vi "Build Board Map.vi"(1 "Map":string="        ...#\n        .#..\n        #...\n        ....\n...#.......#\n........#...\n..#....#....\n..........#.\n        ...#....\n        .....#..\n        .#......\n        ......#.") -> (0 "Board Map":T1[][](array[typedef]) items=["Empty", "Portal", "Open", "Wall", ">", "<", ">-^", ">-v", "^-<", "v-<"])   [LabVIEW 2020, in "AoC 2022.lvlib"]
uses:
  AoC 2022.lvlib
  Map Tile.ctl
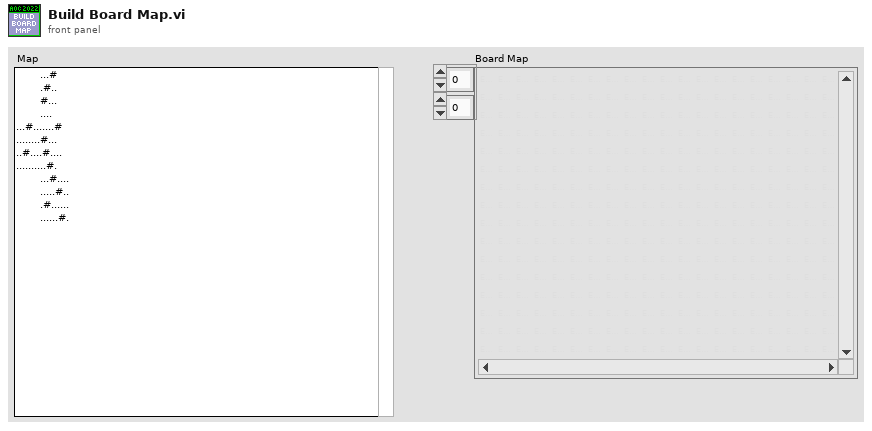
[diagram p1: front panel]
types:
  T1 = typedef "AoC 2022.lvlib/Map Tile.ctl" = u16
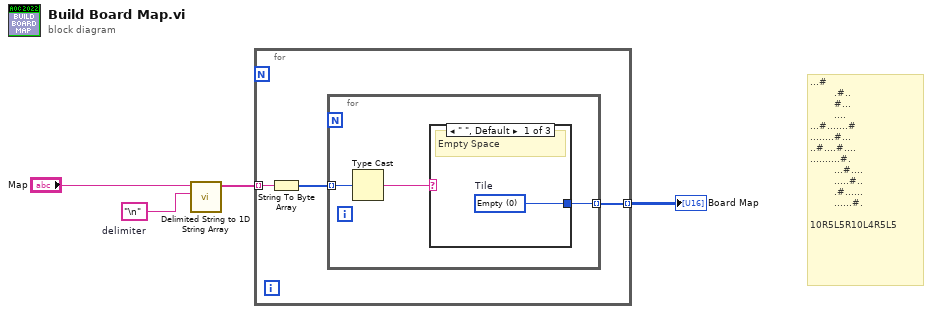
[diagram p0: block diagram]
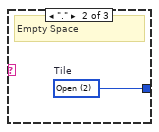
[diagram p2: hidden frame]
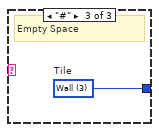
[diagram p3: hidden frame]
diagram:
  w2 = "\n"  # delimiter
  # "...#\n        .#..\n        #...\n        ....\n...#.......#\n........#...\n..#....#....\n..........#.\n        ...#....\n        .....#..\n        .#......\n        ......#.\n\n10R5L5R10L4R5L5"
  n1 = call <vilib>:"Delimited String to 1D String Array.vi"("delimiter"=w2, "delimited string"="Map") -> ("string array"=w3:string[])  [unwired: 9 in]
  n2 = for {
    tunnel: w3 -> [w7] mode=indexing
    tunnel: [w5] -> w4 mode=indexing
    n3 = String To Byte Array(string=w7) -> (unsigned byte array=w6:u8[])
    n4 = for {
      tunnel: w6 -> [w10] mode=indexing
      tunnel: [w8] -> w5 mode=indexing
      n5 = Type Cast(x=w10) -> (*(type *) &x=w9:string)  [unwired: 1 in]
      n6 = case shown="\" \", Default" w9 {
        tunnel: [w11 w12 w13] -> w8
        frame " ", Default {
          w11 = T1 0 items=["Empty", "Portal", "Open", "Wall", ">", "<", ">-^", ">-v", "^-<", "v-<"]  # Tile
          # "Empty Space"
        }
        frame "." {
          w12 = T1 2 items=["Empty", "Portal", "Open", "Wall", ">", "<", ">-^", ">-v", "^-<", "v-<"]  # Tile
          # "Empty Space"
        }
        frame "#" {
          w13 = T1 3 items=["Empty", "Portal", "Open", "Wall", ">", "<", ">-^", ">-v", "^-<", "v-<"]  # Tile
          # "Empty Space"
        }
      }
    }
  }
  "Board Map" <- w4
